vi "Open.vi"(8 "Error In":errorcluster, 11 "Adept Device":u16(xcontrol)) -> (0 "Error Out":errorcluster, 3 "Adept Config":T1)   [LabVIEW 2011, in "LVH-Adept.lvlib"]
doc: "Open a connection to a Digilent FPGA board."
uses:
  LVH-Adept.lvlib
  Private/Type Defs/Device Config.ctl
  Private/Type Defs/Status.ctl
  Private/Type Defs/Adept Device Ctl.xctl
  Private/DMGR/DMGR.lvlib
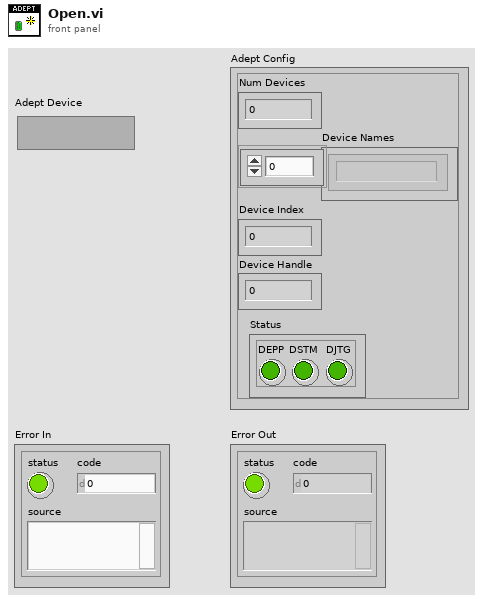
[diagram p1: front panel]
types:
  T1 = typedef "LVH-Adept.lvlib/Device Config.ctl" = cluster{"Num Devices":i32, "Device Names":string[], "Device Index":u16, "Device Handle":u32, "Status":T2}
  T2 = typedef "LVH-Adept.lvlib/Status.ctl" = cluster{"DEPP":bool, "DSTM":bool, "DJTG":bool}
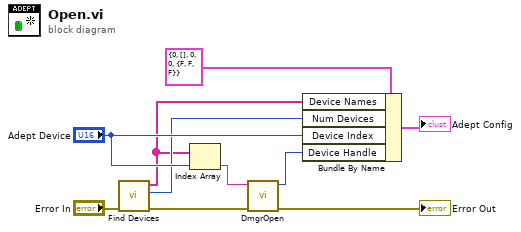
[diagram p0: block diagram]
diagram:
  n1 = call "Find Devices.vi"("Error In"="Error In") -> ("Error Out"=w8:errorcluster, "Num Devices"=w2:i32, "Device Names"=w1:string[])  [unwired: 8 in]
  n2 = Index Array(array=w1, index="Adept Device") -> (element=w9:string)
  n3 = call "DmgrOpen.vi"("Error In"=w8, "Device Name"=w9) -> ("Error Out"=→"Error Out":errorcluster, "Device Handle"=w3:u32)  [unwired: 8 in]
  n4 = Bundle By Name(cluster=T1 {"Num Devices"=0, "Device Names"=[], "Device Index"=0, "Device Handle"=0, "Status"={"DEPP"=FALSE, "DSTM"=FALSE, "DJTG"=FALSE}} ("Adept Config"), "Device Names"=w1, "Num Devices"=w2, "Device Index"="Adept Device", "Device Handle"=w3) -> (→"Adept Config":T1)
